vi "Stop.vi"(8 "error in (no error)":errorcluster, 11 "NI Galvo in":refnum<class "A7M20.lvclass">) -> (0 "error out":errorcluster, 3 "NI Galvo out":refnum<class "A7M20.lvclass">)   [LabVIEW 2015, in "A7M20.lvclass"]
uses:
  A7M20.lvclass
  A7M20.lvclass/A7M20.ctl
  Galvo.lvclass
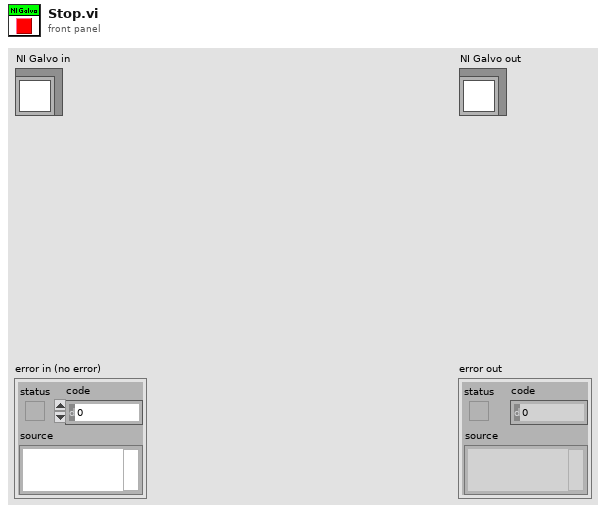
[diagram p1: front panel]
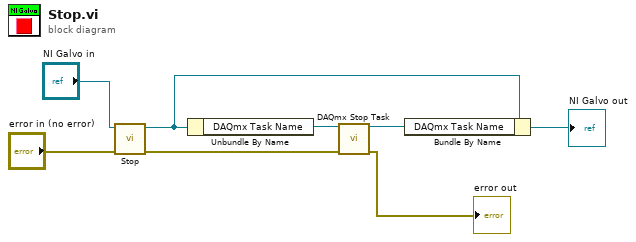
[diagram p0: block diagram]
diagram:
  n1 = call-parent "Stop.vi"("error in (no error)"="error in (no error)", "Galvo in"="NI Galvo in") -> ("error out"=w5:errorcluster, "Galvo out"=w3:refnum<class "A7M20.lvclass">)  [unwired: 8 in]
  n2 = Unbundle By Name(w3) -> ("DAQmx Task Name"=w6:refnum<k21>)
  n3 = call <vilib>:"DAQmx Stop Task.vi"("task/channels in"=w6, "error in"=w5) -> ("task out"=w4:refnum<k21>, "error out"=→"error out":errorcluster)  [unwired: 12 in]
  n4 = Bundle By Name(cluster=w3, "DAQmx Task Name"=w4) -> (→"NI Galvo out":refnum<class "A7M20.lvclass">)
